vi "ziDiscoveryListDevices.vi"(8 "Error In":errorcluster, 11 "ziHandle In":T1 {"Handle" format="0x%08x"; "Conn" format="0x%08x"}) -> (0 "Error Out":errorcluster, 1 "DevicesList":string[](array[string]), 3 "ziHandle Out":T1 {"Handle" format="0x%08x"; "Conn" format="0x%08x"})   [LabVIEW 2018, in "Zurich Instruments LabOne.lvlib"]
doc: "Lists All Devices which are discoverable."
uses:
  Zurich Instruments LabOne.lvlib
  <instrlib>/Zurich Instruments LabOne/Private/ziLV64.framework
  ziTypeHandle.ctl
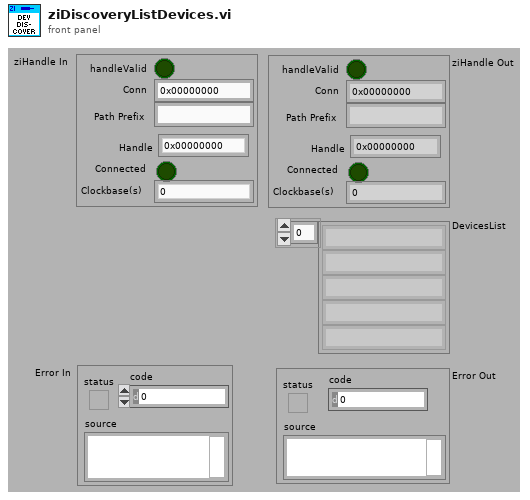
[diagram p1: front panel]
types:
  T1 = typedef "Zurich Instruments LabOne.lvlib/ziTypeHandle.ctl" = cluster{"handleValid":bool, "Conn":u64, "Path Prefix":string, "Handle":u64, "Connected":bool, "Clockbase(s)":dbl}
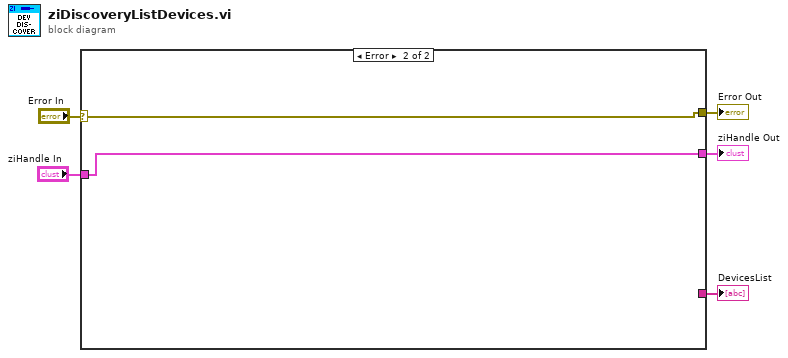
[diagram p0: block diagram]
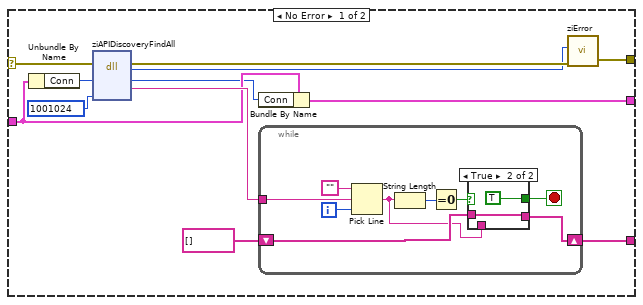
[diagram p2: hidden frame]
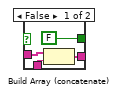
[diagram p3: hidden frame]
diagram:
  n1 = case shown="Error" "Error In" {
    selector: "Error In" -> [w17 w34]
    tunnel: [w14 w34] -> w4
    tunnel: [w10 _] -> w3
    tunnel: "ziHandle In" -> [w8 w33]
    tunnel: [w6 w33] -> w1
    frame No Error {
      n2 = Unbundle By Name(w8) -> ("Conn"=w9:u64)
      n3 = dll-call lib="Applications/National Instruments/LabVIEW 2019 64-bit/instr.lib/Zurich Instruments LabOne/Private/ziLV*.*" fn="ziAPIDiscoveryFindAll"(error in=w17, "conn"=w9, "Buffer"=u32 1001024 ("arg2")) -> (error out=w16:errorcluster, "return type"=w15:u32, "conn"=w7:u64, "DevicesList"=w12:string)  [unwired: 4 in, 1 out]
      n4 = Bundle By Name(cluster=w8, "Conn"=w7) -> (w6:T1)
      n5 = while {
        shift-right: [w19] -> w10
        shift-left: string[] [] -> [w20]
        tunnel: w12 -> [w22]
        i -> [w26]
        stop <- w21 stop-if-true
        n6 = Pick Line(string ("")="", multi-line string=w22, line index=w26) -> (output string=w18:string)
        n7 = String Length(string=w18) -> (length=w24:i32)
        n8 = Equal To 0?(x=w24) -> (x = 0?=w23:bool)
        n9 = case shown="True" w23 {
          tunnel: [FALSE TRUE] -> w21
          tunnel: w20 -> [w29 w31]
          tunnel: [w28 w31] -> w19
          tunnel: w18 -> [w27 _]
          frame False {
            n10 = Build Array (concatenate)(w29, w27) -> (w28:string[])
          }
          frame True {
          }
        }
      }
      n11 = call "ziError.vi"("ziErrorCode"=w15, "Error In"=w16) -> ("Error Out"=w14:errorcluster)  [unwired: 3 in, 1 out]
    }
    frame Error {
    }
  }
  "Error Out" <- w4
  "DevicesList" <- w3
  "ziHandle Out" <- w1
